vi "Manual_Control_Main.vi"() -> ()   [LabVIEW 2024]
uses:
  <vilib>/Platform/TimedLoop/XDataNode/timing_clust.ctl
  <vilib>/Platform/TimedLoop/XDataNode/nitl_modes.ctl
  <vilib>/Platform/TimedLoop/XDataNode/wakeup.ctl
  <vilib>/addons/Maxon Motor/EPOS2 CANopen/CANopen/sbCANopenBaseClass.lvclass
  <vilib>/platform/TimedLoop/XDataNode/XDataNode.xnode
  <vilib>/Platform/TimedLoop/XDataNode/XDNodeRunTimeDep.lvlib
panel:
  out "ResetPID":bool
  in  "Motor_index":i32[](array[numeric])=[3, 6, 9, 12, 2, 7, 8, 13, 4, 5, 10, 11, 1, 14]
  out "canERROR":errorcluster[][](array[cluster])
  in  "Control Mode":string="O"
  in  "goal_Tensions":dbl[](array[numeric])=[0.0, 0.0, 0.0, 0.0, 0.0, 0.0, 0.0, 0.0, 0.0, 0.0, 0.0, 0.0, 0.0, 0.0]
  in  "TARE":bool
  in  "curr_Tensions":dbl[](array[numeric])
  out "DAQ Error":errorcluster
  out "Write Late?":bool
  out "Write Time [us]":i64
  in  "Tare_Tensions":dbl[](array[numeric])=[1.6875269817998764, 0.7228096971601798, 1.962272927280566, 2.6696462364433735, 2.7003690389898463, 3.088938448864716, 1.6430905755314908, 3.0754139877790347, 3.5546581214666455, 3.2737863413382597, 4.727265898547672, 2.6001067118162604, 1.980007529135911, 1.8614502099489874]
  in  "STOP CONTROLLER":bool
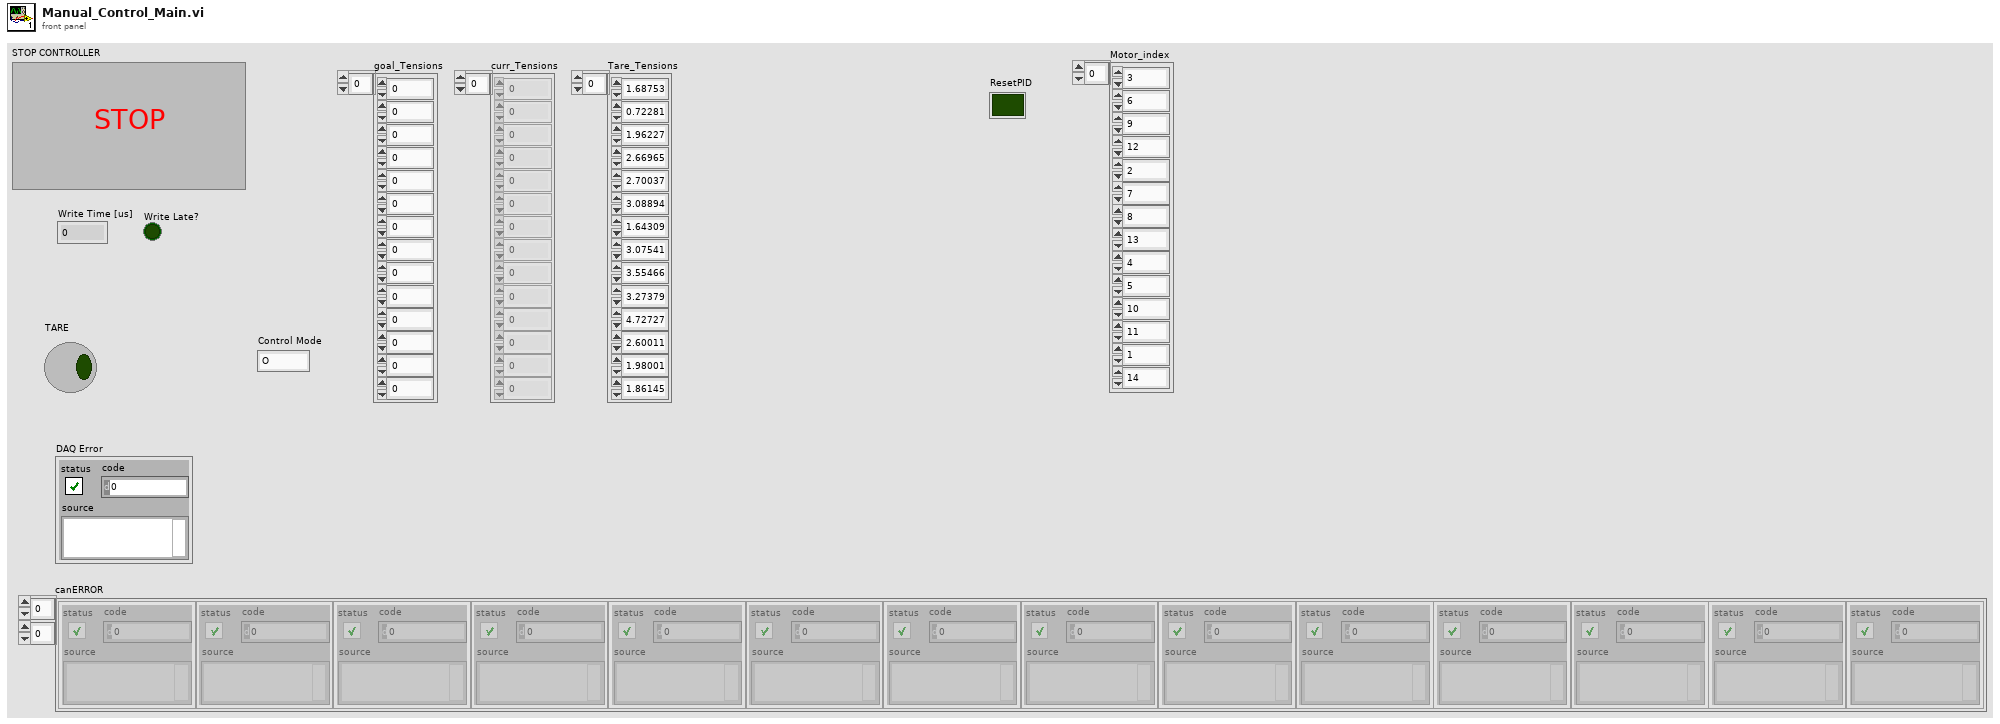
[diagram p1: front panel]
types:
  T1 = typedef "XDNodeRunTimeDep.lvlib/timing_clust.ctl" = cluster{"Expected End [f-1]":u64, "Actual End [f-1]":u64, "Finished Late? [f-1]":bool, "Expected End [i-1]":u64, "Actual End [i-1]":u64, "Finished Late? [i-1]":bool, "Expected Start [i]":u64, "Actual Start [i]":u64, "Expected Start [f]":u64, "Actual Start [f]":u64, "Source Name":string, "Structure Name":string, "Period":i64, "Deadline":i64, "Offset":i64, "Start":i64, "Priority":i32, "Timeout":i32, "Mode":T2, "Wakeup Reason":T3, "Error":errorcluster, "Source Type":string, "Secondary Source Type":string, "Global End Time":u64, "Global Start Time":u64, "Frame Duration":u64, "Iteration Duration":u64, "Assigned CPU":i32, "I/O Scan Engine Mode":u32}
  T2 = typedef "XDNodeRunTimeDep.lvlib/nitl_modes.ctl" = enum32{"No Change", "Process missed periods, maintain original phase", "Discard missed periods, maintain original phase", "Process missed periods, ignore original phase", "Discard missed periods, ignore original phase"}
  T3 = typedef "XDNodeRunTimeDep.lvlib/wakeup.ctl" = enum32{"Normal", "Aborted", "Asynchronous wakeup", "Timing source error", "Timed loop error", "Timeout"}
  T4 = cluster{"curr_Tensions":dbl[], "goal_Tensions":dbl[]}
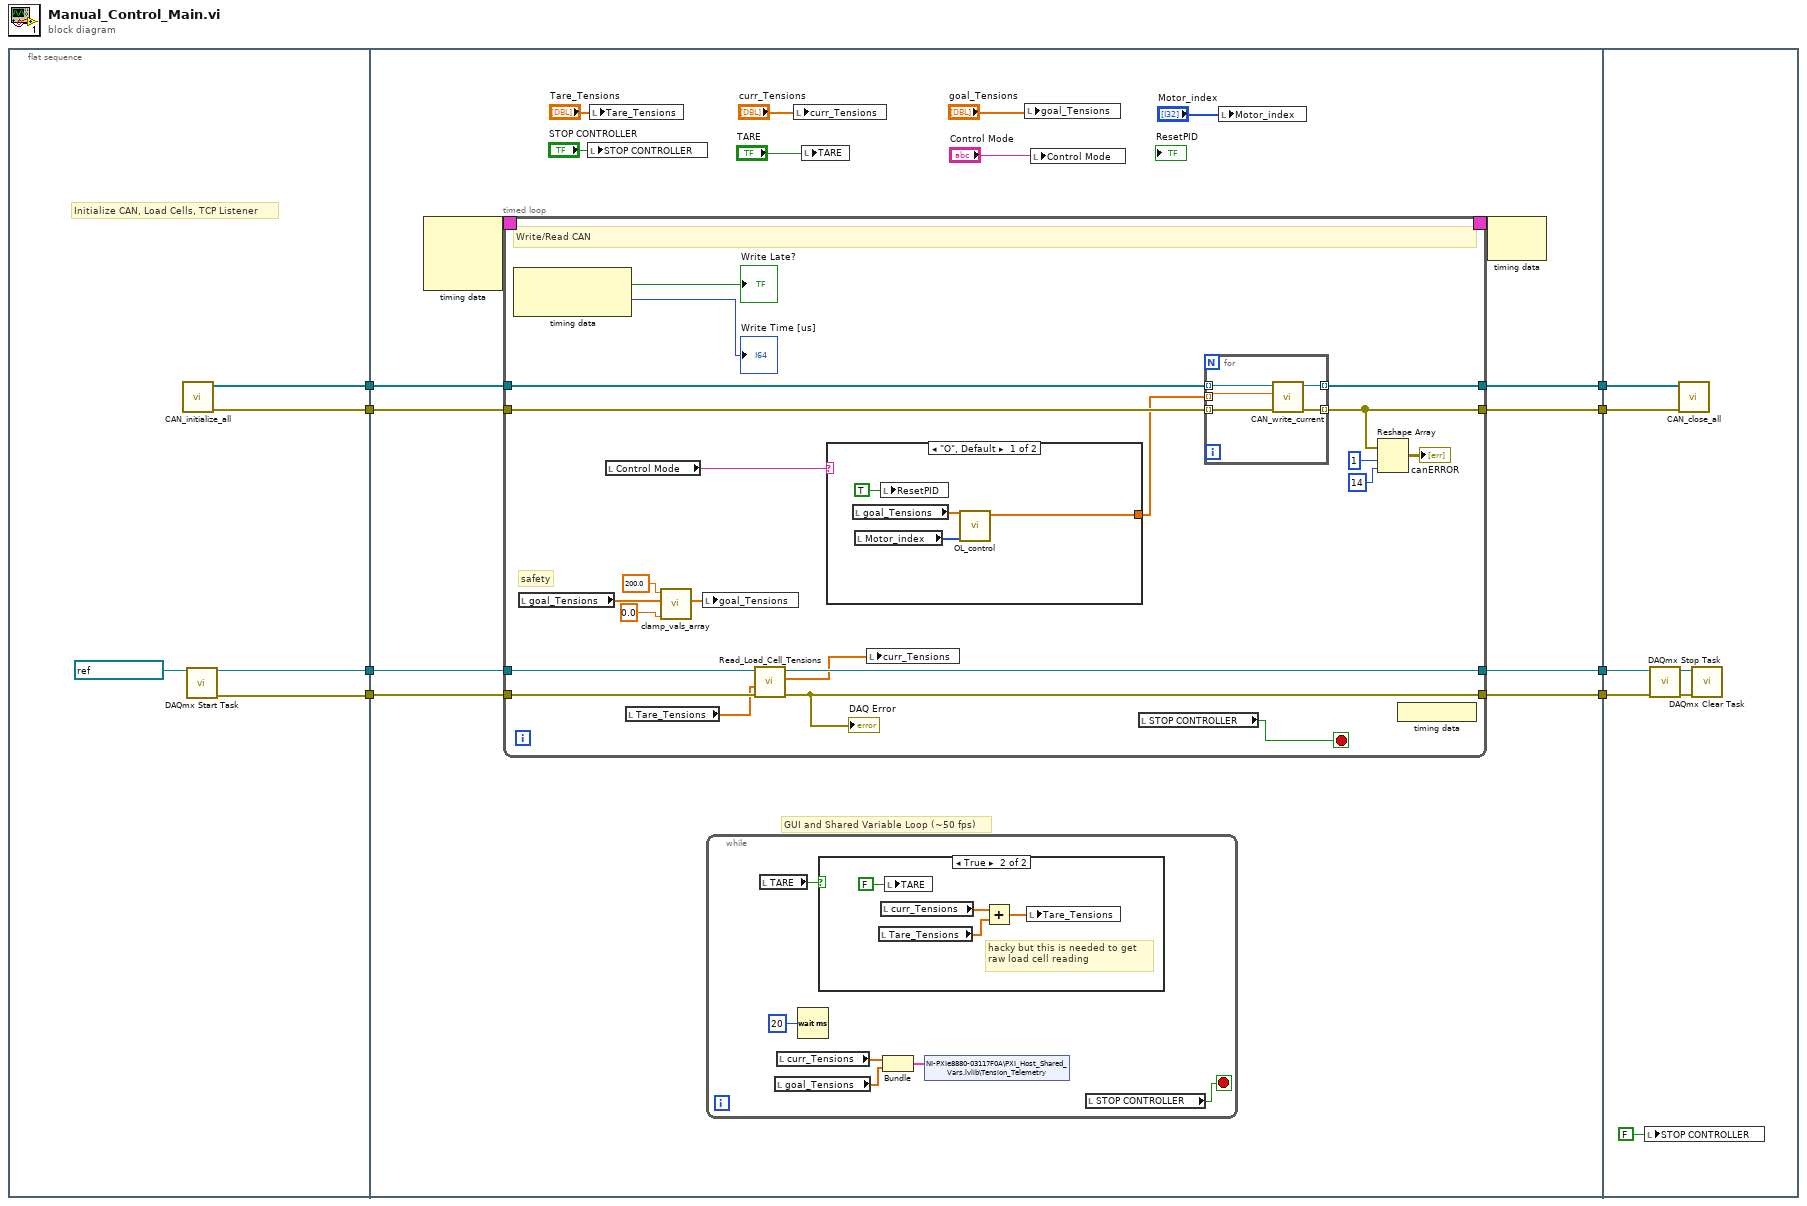
[diagram p0: block diagram]
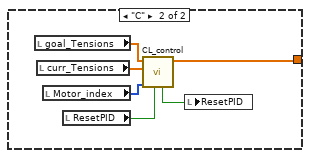
[diagram p3: hidden frame]
diagram:
  n1 = flat-sequence {
    tunnel: [w12] -> w8
    tunnel: [w13] -> w7
    tunnel: [w9] -> w4
    tunnel: [w10] -> w3
    tunnel: w8 -> [w28]
    tunnel: w7 -> [w27]
    tunnel: [w26] -> w6
    tunnel: [w25] -> w5
    tunnel: w4 -> [w23]
    tunnel: w3 -> [w22]
    tunnel: [w21] -> w2
    tunnel: [w20] -> w1
    tunnel: w6 -> [w90]
    tunnel: w5 -> [w89]
    tunnel: w2 -> [w86]
    tunnel: w1 -> [w85]
    frame #0 {
      # "Initialize CAN, Load Cells, TCP Listener"
      n2 = call "CAN_initialize_all.vi"() -> ("Array of Canopen Sessions"=w13:refnum<class "sbCANopenBaseClass.lvclass">[], "Array of Error out's"=w12:errorcluster[])  [unwired: 5 in]
      n3 = call <vilib>:"DAQmx Start Task.vi"("task/channels in"=refnum<k21> "SCI_TenSen") -> ("task out"=w9:refnum<k21>, "error out"=w10:errorcluster)  [unwired: 13 in]
    }
    frame #1 {
      # "GUI and Shared Variable Loop (~50 fps)"
      n4 = node-c288() -> (w30:T1)  [unwired: 3 in]
      n5 = timed-loop {
        tunnel: w28 -> [w54]
        tunnel: [w46] -> w26
        timing: w30 -> [_]
        timing-out: [_] -> w29
        tunnel: w27 -> [w55]
        tunnel: [w59] -> w25
        tunnel: w23 -> [w58]
        tunnel: w22 -> [w57]
        tunnel: [w56] -> w21
        tunnel: [w53] -> w20
        stop <- w60 stop-if-true
        # "safety"
        # "Write/Read CAN"
        n6 = node-c288() -> (→"Write Late?":bool, →"Write Time [us]":i64)  [unwired: 1 in]
        n7 = local read "goal_Tensions"() -> (w41:dbl[])
        n8 = local read "Control Mode"() -> (w51:string)
        n9 = local read "Tare_Tensions"() -> (w52:dbl[])
        n10 = call "clamp_vals_array.vi"("Min Val"=0.0, "Input Array"=w41, "Max Val"=200.0) -> ("Output Array"=w42:dbl[])  [unwired: 8 in]
        n11 = local write "goal_Tensions"(w42) -> ()
        n12 = call "Read_Load_Cell_Tensions.vi"("error in (no error)"=w57, "Tare Tension"=w52, "Refnum in"=w58) -> ("error out"=w53:errorcluster, "Measured Cable Tensions"=w50:dbl[], "Refnum out"=w56:refnum<k21>)  [unwired: 4 in]
        "DAQ Error" <- w53
        n13 = case shown="\"O\", Default" w51 {
          tunnel: [w66 w72] -> w49
          frame "O", Default {
            n14 = local read "goal_Tensions"() -> (w63:dbl[])
            n15 = local read "Motor_index"() -> (w65:i32[])
            n16 = local write "ResetPID"(TRUE) -> ()
            n17 = call "OL_control.vi"("Motor_index"=w65, "goal_Tensions"=w63) -> ("can_Current"=w66:dbl[])  [unwired: 9 in]
          }
          frame "C" {
            n18 = local read "goal_Tensions"() -> (w67:dbl[])
            n19 = local read "curr_Tensions"() -> (w68:dbl[])
            n20 = local read "Motor_index"() -> (w71:i32[])
            n21 = local read "ResetPID"() -> (w70:bool)
            n22 = call "CL_control.vi"("ResetPID"=w70, "Motor_index"=w71, "curr_Tensions"=w68, "goal_Tensions"=w67) -> ("can_Current"=w72:dbl[], "Reset PID (output)"=w69:bool)  [unwired: 6 in]
            n23 = local write "ResetPID"(w69) -> ()
          }
        }
        n24 = local write "curr_Tensions"(w50) -> ()
        n25 = local read "STOP CONTROLLER"() -> (w60:bool)
        n26 = for {
          tunnel: [w74] -> w59 mode=indexing
          tunnel: [w75] -> w46 mode=indexing
          tunnel: w55 -> [w77] mode=indexing
          tunnel: w54 -> [w76] mode=indexing
          tunnel: w49 -> [w73] mode=indexing
          n27 = call "CAN_write_current.vi"("error in"=w76, "Current Command [mA]"=w73, "CANopen Session In"=w77) -> ("error out"=w75:errorcluster, "CANopen Session Out"=w74:refnum<class "sbCANopenBaseClass.lvclass">)  [unwired: 7 in]
        }
        n28 = Reshape Array(w46, 1 ("dimension size"), 14 ("dimension size")) -> (→"canERROR":errorcluster[][])
        n29 = node-c288() -> ()  [unwired: 1 out]
      }
      n30 = local write "STOP CONTROLLER"("STOP CONTROLLER") -> ()
      n31 = local write "Tare_Tensions"("Tare_Tensions") -> ()
      n32 = while {
        stop <- w36 stop-if-true
        n33 = local read "TARE"() -> (w35:bool)
        n34 = local read "goal_Tensions"() -> (w31:dbl[])
        n35 = local read "curr_Tensions"() -> (w34:dbl[])
        n36 = Wait (ms)(milliseconds to wait=u32 20) -> ()  [unwired: 1 out]
        n37 = case shown="True" w35 {
          frame False {
          }
          frame True {
            # "hacky but this is needed to get \nraw load cell reading"
            n38 = local read "Tare_Tensions"() -> (w38:dbl[])
            n39 = local read "curr_Tensions"() -> (w39:dbl[])
            n40 = local write "TARE"(FALSE ("TARE")) -> ()
            n41 = Add(x=w39, y=w38) -> (x+y=w40:dbl[])
            n42 = local write "Tare_Tensions"(w40) -> ()
          }
        }
        n43 = Bundle("curr_Tensions"=w34, "goal_Tensions"=w31) -> (w33:T4)  [unwired: 1 in]
        n44 = shared-variable "NI-PXIe8880-03117F0A\\PXI_Host_Shared_Vars.lvlib\\Tension_Telemetry"(w33) -> ()  [unwired: 1 in, 1 out]
        n45 = local read "STOP CONTROLLER"() -> (w36:bool)
      }
      n46 = local write "curr_Tensions"("curr_Tensions") -> ()
      n47 = local write "TARE"("TARE") -> ()
      n48 = local write "goal_Tensions"("goal_Tensions") -> ()
      n49 = local write "Control Mode"("Control Mode") -> ()
      n50 = local write "Motor_index"("Motor_index") -> ()
      n51 = node-c288(w29) -> ()  [unwired: 1 out]
    }
    frame #2 {
      n52 = local write "STOP CONTROLLER"(FALSE ("STOP CONTROLLER")) -> ()
      n53 = call <vilib>:"DAQmx Stop Task.vi"("task/channels in"=w86, "error in"=w85) -> ("task out"=w87:refnum<k21>, "error out"=w88:errorcluster)  [unwired: 12 in]
      n54 = call "CAN_close_all.vi"("Input Error out array"=w90, "Input CANopen Sessions array"=w89) -> ()  [unwired: 10 in]
      n55 = call <vilib>:"DAQmx Clear Task.vi"("task in"=w87, "error in"=w88) -> ()  [unwired: 13 in, 1 out]
    }
  }
